vi "KE3706A_CommandsGlobal.vi"() -> ()   [LabVIEW 2013, in "KE3706A.lvclass"]
uses:
  KE3706A.lvclass
panel:
  in  "Keithley 3706A Switching GPIB Setup":T1={"Instrument name"="Pickering Matrix", "Instrument type"=2, "Command \"Matrix Reset\""="areset %s", "Command \"Connect MUX Channel\""="mclose %s,%d,%d", "Command \"Disconnect Matrix Channels\""="mopen %s,%d,%d", "Mux1 slot"="4", "Mux2 slot"="5"} {"Instrument type" items=["Supply", "LCR", "Switching"]}
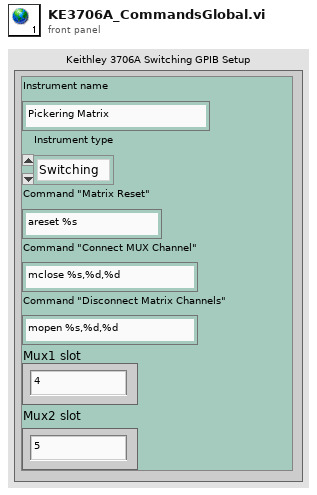
[diagram p1: front panel]
types:
  T1 = cluster{"Instrument name":string, "Instrument type":u16, "Command \"Matrix Reset\"":string, "Command \"Connect MUX Channel\"":string, "Command \"Disconnect Matrix Channels\"":string, "Mux1 slot":string, "Mux2 slot":string}
diagram:
